vi "HSMS Stop.vi"(8 "error in (no error)":errorcluster, 11 "HSMS Class in":refnum<class "HSMS Class.lvclass">) -> (0 "error out":errorcluster, 3 "HSMS Class out":refnum<class "HSMS Class.lvclass">)   [LabVIEW 2020, in "SECS Communication.lvlib" / "HSMS Class.lvclass"]
uses:
  HSMS Class.lvclass
  HSMS Class.lvclass/HSMS Class.ctl
  Read Alive Notifier.vi
  Read Listener Refnum.vi
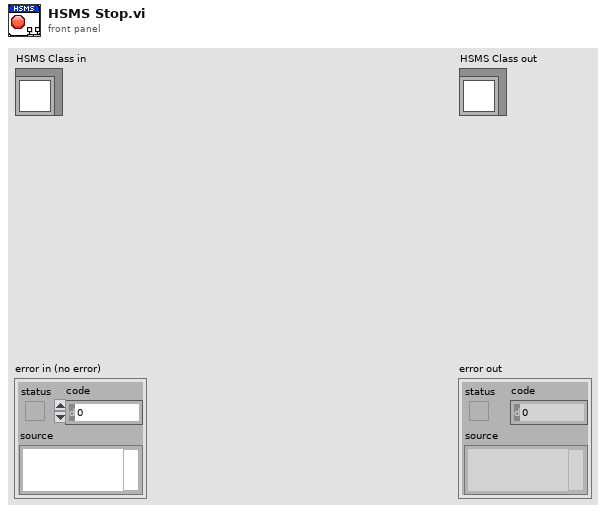
[diagram p1: front panel]
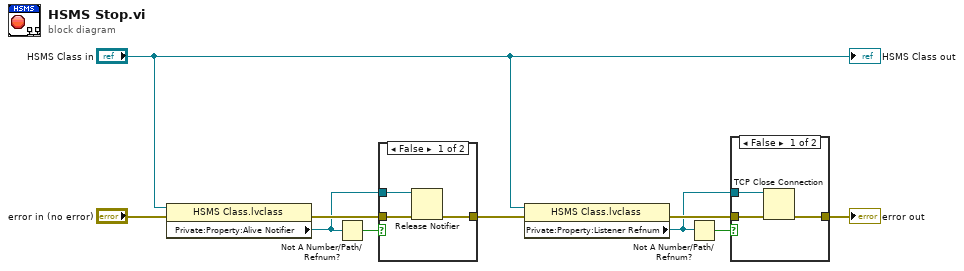
[diagram p0: block diagram]
diagram:
  n1 = property class="HSMS Class.lvclass"(reference="HSMS Class in", error in="error in (no error)") -> (error out=w8:errorcluster, "Private:Property:Alive Notifier"=w7:refnum<notifier>)  [unwired: 1 out]
  n2 = Not A Number/Path/Refnum?(number/path/refnum=w7) -> (NaN/Path/Refnum?=w10:bool)
  n3 = case shown="False" w10 {
    tunnel: w8 -> [w12 w14]
    tunnel: w7 -> [w13 _]
    tunnel: [w11 w14] -> w4
    frame False {
      n4 = Release Notifier(notifier=w13, error in (no error)=w12) -> (error out=w11:errorcluster)  [unwired: 1 in, 2 out]
    }
    frame True {
    }
  }
  n5 = property class="HSMS Class.lvclass"(reference="HSMS Class in", error in=w4) -> (error out=w2:errorcluster, "Private:Property:Listener Refnum"=w1:refnum<k5>)  [unwired: 1 out]
  n6 = Not A Number/Path/Refnum?(number/path/refnum=w1) -> (NaN/Path/Refnum?=w6:bool)
  n7 = case shown="False" w6 {
    tunnel: w2 -> [w16 w18]
    tunnel: w1 -> [w17 _]
    tunnel: [w15 w18] -> w5
    frame False {
      n8 = TCP Close Connection(connection ID=w17, error in (no error)=w16) -> (error out=w15:errorcluster)  [unwired: 1 in, 1 out]
    }
    frame True {
    }
  }
  "error out" <- w5
  "HSMS Class out" <- "HSMS Class in"
